vi "Template - DMM Acquire Multiple.vi"() -> ()   [LabVIEW 2013]
doc: "This example shows how to configure a measurement and take multiple readings."
uses:
  <instrlib>/_Template - DMM/Public/Data/Read (Multiple Points).vi
  <instrlib>/_Template - DMM/Template - DMM.lvlib
panel:
  in  "Serial Configuration":T1={"Baud Rate"=9600, "Parity"=0, "Data Bits"=7, "Stop Bits"=10, "Flow Control"=0} {"Flow Control" items=["None", "XON/XOFF", "RTS/CTS", "XON/XOFF & RTS/CTS", "DTR/DSR", "XON/XOFF & DTR/DSR"]; "Stop Bits" items=["1.0"=10, "1.5"=15, "2.0"=20]; "Data Bits" items=["7"=7, "8"=8]; "Parity" items=["None", "Odd", "Even", "Mark", "Space"]; "Baud Rate" items=["300"=300, "600"=600, "1200"=1200, "2400"=2400, "4800"=4800, "9600"=9600, "19200"=19200]}
  out "Measurements":dbl[](array[numeric])
  in  "Timeout (10000 ms)":i32=10000 format="%#.6g"
  in  "Sample Count (25)":i32=25
  in  "Function (0: DC Volts)":u16(ring) items=["DC Volts", "AC Volts", "DC Current", "AC Current", "2-Wire Resistance", "4-Wire Resistance", "Temperature", "Frequency", "Period", "Continuity", "Diode"]
  in  "VISA resource name":refnum<visa-resource-name>
  # "(c) 2007 <Enter Company Name Here>.  ALL RIGHTS RESERVED."
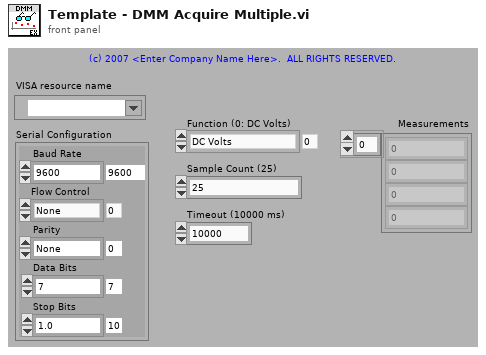
[diagram p1: front panel]
types:
  T1 = cluster{"Baud Rate":u32, "Parity":u16, "Data Bits":u16, "Stop Bits":u16, "Flow Control":u16}
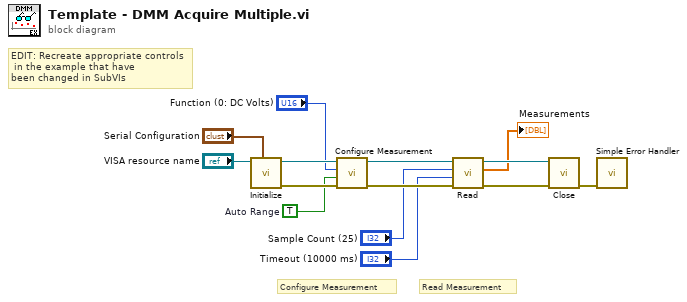
[diagram p0: block diagram]
diagram:
  w10 = TRUE  # Auto Range
  # "EDIT: Recreate appropriate controls\n in the example that have \nbeen changed in SubVIs"
  # "Read Measurement"
  # "Configure Measurement"
  n1 = call <instrlib>:"Initialize.vi"("Serial Configuration"="Serial Configuration", "VISA resource name"="VISA resource name") -> ("error out"=w11:errorcluster, "VISA resource name out"=w12:refnum<visa-resource-name>)  [unwired: 8 in]
  n2 = call <instrlib>:"Configure Measurement.vi"("error in (no error)"=w11, "Auto Range (T:Enable)"=w10, "Function (0: DC Volts)"="Function (0: DC Volts)", "VISA resource name"=w12) -> ("error out"=w8:errorcluster, "VISA resource name out"=w7:refnum<visa-resource-name>)  [unwired: 6 in]
  n3 = call-poly <instrlib>:"Read.vi"("error in (no error)"=w8, "Timeout (10000 ms)"="Timeout (10000 ms)", "Sample Count (1)"="Sample Count (25)", "VISA resource name"=w7) -> ("error out"=w9:errorcluster, "Measurements"=→"Measurements":dbl[], "VISA resource name out"=w6:refnum<visa-resource-name>)  [unwired: 5 in]
  n4 = call <instrlib>:"Close.vi"("error in (no error)"=w9, "VISA resource name"=w6) -> ("error out"=w14:errorcluster)  [unwired: 9 in]
  n5 = call <vilib>:"Simple Error Handler.vi"("error in (no error)"=w14) -> ()  [unwired: 4 in, 5 out]
